vi "find threat.vi"(9 "Team Index":i32, 10 "View":i32[](array[numeric]) caption="View (Team Index, -1: empty)") -> (1 "Enemy Squares":T1[](array[typedef]), 2 "Empty Squares":T1[](array[typedef]), 3 "Friendly Squares":T1[](array[typedef]))   [LabVIEW 2015, in "JFD_Common.lvlib"]
uses:
  JFD_Common.lvlib
  Type Defs/Direction Enum.ctl
  Type Defs/SB Type Defs.lvlib
panel:
  # "NW\nN\nNE\nE\nSE\nS\nSW\nW"
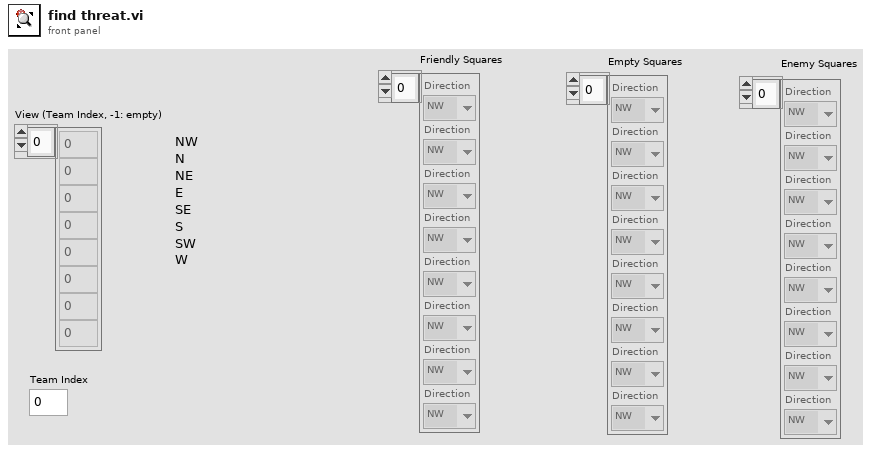
[diagram p1: front panel]
types:
  T1 = typedef "SB Type Defs.lvlib/Direction Enum.ctl" = enum16{"NW", "N", "NE", "E", "SE", "S", "SW", "W"}
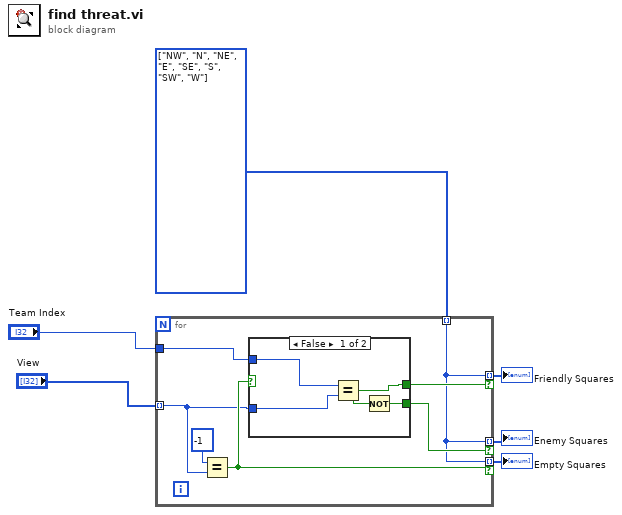
[diagram p0: block diagram]
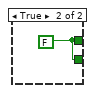
[diagram p2: hidden frame]
diagram:
  w1 = T1[] [enum."NW", enum."N", enum."NE", enum."E", enum."SE", enum."S", enum."SW", enum."W"] items=["NW", "N", "NE", "E", "SE", "S", "SW", "W"] ("Friendly Squares")
  n1 = for {
    tunnel: "View" -> [w7] mode=indexing
    tunnel: [w8] -> w6 mode=indexing if=w9
    tunnel: [w8] -> w5 mode=indexing if=w12
    tunnel: [w8] -> w4 mode=indexing if=w11
    tunnel: "Team Index" -> [w10]
    tunnel: w1 -> [w8] mode=indexing
    n2 = Equal?(x=-1, y=w7) -> (x = y?=w12:bool)
    n3 = case shown="False" w12 {
      tunnel: [w15 w18] -> w11
      tunnel: w7 -> [w17 _]
      tunnel: w10 -> [w16 _]
      tunnel: [w14 w18] -> w9
      frame False {
        n4 = Equal?(x=w16, y=w17) -> (x = y?=w15:bool)
        n5 = Not(x=w15) -> (.not. x?=w14:bool)
      }
      frame True {
        w18 = FALSE
      }
    }
  }
  "Enemy Squares" <- w6
  "Empty Squares" <- w5
  "Friendly Squares" <- w4
